vi "CTRL_Convert serial string to Eng vals.vi"(1 "Serial buffer string (excluding FrameChar)":string) -> (0 "Data":T1)   [LabVIEW 2020]
uses:
  ctls/CTRL_Data_Out.ctl
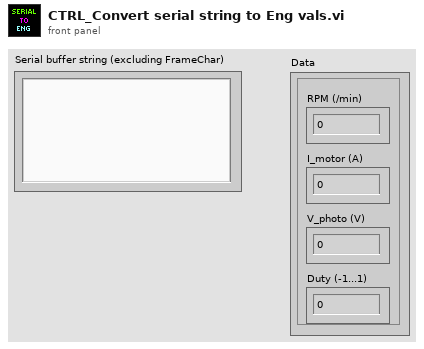
[diagram p1: front panel]
types:
  T1 = typedef "CTRL_Data_Out.ctl" = cluster{"RPM (/min)":sgl, "I_motor (A)":sgl, "V_photo (V)":sgl, "Duty (-1...1)":sgl}
  T2 = cluster{"[0]":sgl, "[1]":sgl, "[2]":sgl, "[3]":sgl}
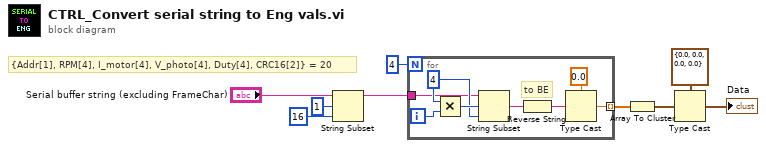
[diagram p0: block diagram]
diagram:
  # "{Addr[1], RPM[4], I_motor[4], V_photo[4], Duty[4], CRC16[2]} = 20"
  n1 = String Subset(string="Serial buffer string (excluding FrameChar)", offset (0)=1, length (rest)=16 ("length (rest)")) -> (substring=w8:string)
  n2 = for {
    N: 4 -> [_]
    tunnel: [w11] -> w4 mode=indexing
    tunnel: w8 -> [w10]
    i -> [w17]
    w15 = 4 ("x")
    # "to BE"
    n3 = Multiply(x=w15, y=w17) -> (x*y=w16:i32)
    n4 = String Subset(string=w10, offset (0)=w16, length (rest)=w15) -> (substring=w14:string)
    n5 = Reverse String(1:w14) -> (0:w13:string)
    n6 = Type Cast(type=sgl 0.0 ("byte count"), x=w13) -> (*(type *) &x=w11:sgl)
  }
  n7 = Array To Cluster(array=w4) -> (cluster=w3:T2)
  n8 = Type Cast(type=T1 {"RPM (/min)"=0.0, "I_motor (A)"=0.0, "V_photo (V)"=0.0, "Duty (-1...1)"=0.0} ("Data"), x=w3) -> (*(type *) &x=→"Data":T1)
